vi "WPI_RobotDriveDoesDevRefExist.vi"(0 "RobotDriveDevRefArray":T1[](array[typedef]), 7 "RobotDriveDevRef":T1={"DevStatus"={"status"=FALSE, "code"=0, "source"=""}, "Motors[]"=[], "Square Inputs"=FALSE, "Max Output"=1.0}) -> (4 "index":i32, 8 "exists":bool)   [LabVIEW 2025]
doc: "This is used to find the index of a DevRef within an array of DevRefs."
uses:
  <vilib>/Rock Robotics/WPI/RobotDrive/WPI_RobotDriveDevRef.ctl
  <vilib>/Rock Robotics/WPI/MotorControl/WPI_MotorControlDeviceRef.ctl
  <vilib>/Rock Robotics/WPI/MotorControl/WPI_MotorControlType.ctl
  <vilib>/Rock Robotics/SystemInterfaces/DIO/FPGA_DIOPWMChannel.ctl
  <vilib>/Rock Robotics/WPI/PWM/WPI_PWMDeadband.ctl
  <vilib>/Rock Robotics/SystemInterfaces/DIO/FPGA_DIOChannel.ctl
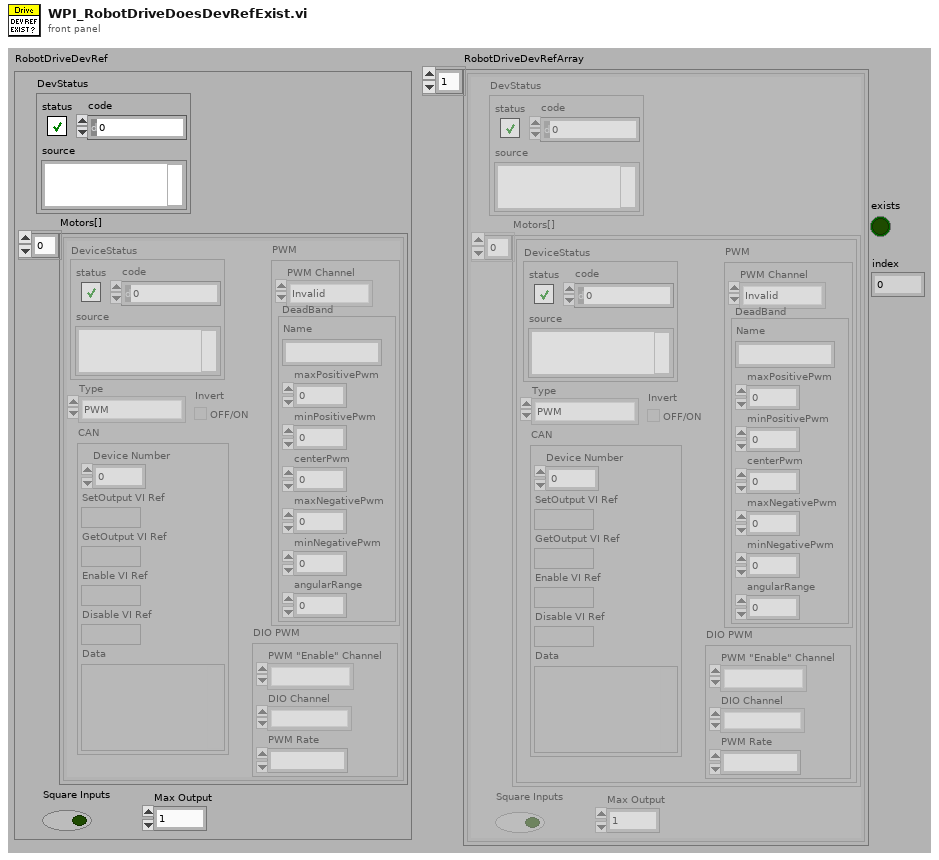
[diagram p1: front panel]
types:
  T1 = typedef "WPI_RobotDriveDevRef.ctl" = cluster{"DevStatus":errorcluster, "Motors[]":T2[], "Square Inputs":bool, "Max Output":dbl}
  T2 = typedef "WPI_MotorControlDeviceRef.ctl" = cluster{"DeviceStatus":errorcluster, "Type":T3, "PWM":cluster{"PWM Channel":T4, "DeadBand":T5}, "CAN":cluster{"Device Number":u8, "SetOutput VI Ref":variant, "GetOutput VI Ref":variant, "Enable VI Ref":variant, "Disable VI Ref":variant, "Data":variant}, "Invert":bool, "DIO PWM":cluster{"PWM \"Enable\" Channel":T4, "DIOChannel":T6, "PWM Rate":dbl}}
  T3 = typedef "WPI_MotorControlType.ctl" = enum16{"PWM", "CAN", "DIO PWM"}
  T4 = typedef "FPGA_DIOPWMChannel.ctl" = enum8{"PWM 0", "PWM 1", "PWM 2", "PWM 3", "PWM 4", "PWM 5", "PWM 6", "PWM 7", "PWM 8", "PWM 9", "PWM MXP 0", "PWM MXP 1", "PWM MXP 2", "PWM MXP 3", "PWM MXP 4", "PWM MXP 5", "PWM MXP 6", "PWM MXP 7", "PWM MXP 8", "PWM MXP 9", "Invalid"}
  T5 = typedef "WPI_PWMDeadband.ctl" = cluster{"Name":string, "maxPositivePwm":i32, "minPositivePwm":i32, "centerPwm":i32, "maxNegativePwm":i32, "minNegativePwm":i32, "angularRange":u16}
  T6 = typedef "FPGA_DIOChannel.ctl" = enum8{"DIO 0", "DIO 1", "DIO 2", "DIO 3", "DIO 4", "DIO 5", "DIO 6", "DIO 7", "DIO 8", "DIO 9", "DIO MXP 0", "DIO MXP 1", "DIO MXP 2", "DIO MXP 3", "DIO MXP 4", "DIO MXP 5", "DIO MXP 6", "DIO MXP 7", "DIO MXP 8", "DIO MXP 9", "DIO MXP 10", "DIO MXP 11", "DIO MXP 12", "DIO MXP 13", "DIO MXP 14", "DIO MXP 15", "SPI Port CS1", "SPI Port CS2", "SPI Port CS3", "SPI Port MISO", "SPI Port MOSI", "Invalid"}
  T7 = cluster{"[0]":T4, "[1]":T4, "[2]":T4, "[3]":T4, "[4]":T4, "[5]":T4, "[6]":T4, "[7]":T4, "[8]":T4}
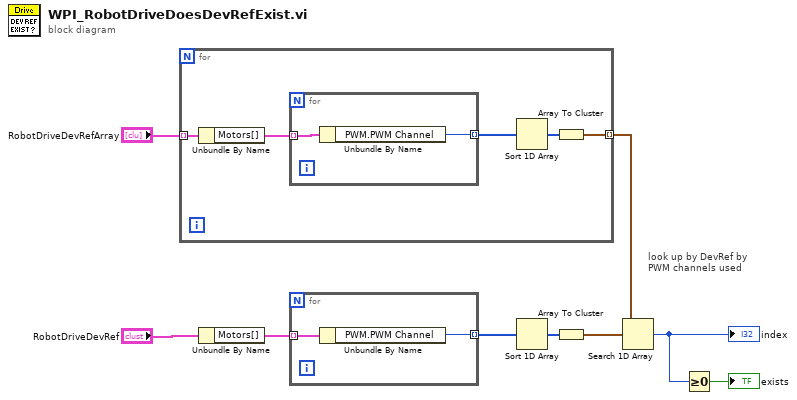
[diagram p0: block diagram]
diagram:
  # "look up by DevRef by PWM channels used"
  n1 = for {
    tunnel: "RobotDriveDevRefArray" -> [w12] mode=indexing
    tunnel: [w10] -> w5 mode=indexing
    n2 = Unbundle By Name(w12) -> ("Motors[]"=w13:T2[])
    n3 = for {
      tunnel: w13 -> [w16] mode=indexing
      tunnel: [w15] -> w14 mode=indexing
      n4 = Unbundle By Name(w16) -> ("PWM.PWM Channel"=w15:T4)
    }
    n5 = Sort 1D Array(array=w14) -> (sorted array=w11:T4[])
    n6 = Array To Cluster(array=w11) -> (cluster=w10:T7)
  }
  n7 = Unbundle By Name("RobotDriveDevRef") -> ("Motors[]"=w8:T2[])
  n8 = for {
    tunnel: w8 -> [w18] mode=indexing
    tunnel: [w17] -> w7 mode=indexing
    n9 = Unbundle By Name(w18) -> ("PWM.PWM Channel"=w17:T4)
  }
  n10 = Sort 1D Array(array=w7) -> (sorted array=w2:T4[])
  n11 = Array To Cluster(array=w2) -> (cluster=w1:T7)
  n12 = Search 1D Array(1D array=w5, element=w1) -> (index of element=w3:i32)  [unwired: 1 out]
  "index" <- w3
  n13 = Greater Or Equal To 0?(x=w3) -> (x >= 0?=→"exists":bool)
